vi "Reports.Find Image File Objs Based on Data File Path.vi"(10 "Pattern":string="png", 11 "Data File":path) -> (3 "FIle Objs":T1[](array[typedef]))   [LabVIEW 2018]
uses:
  Report.Result FileDataObject.ctl
  <vilib>/KATE/Files/File Utils.lvlib
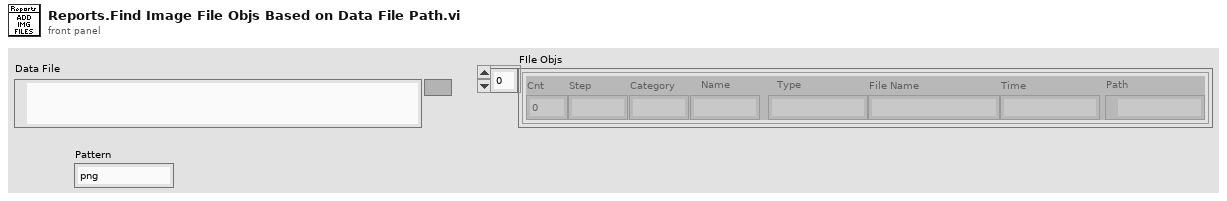
[diagram p1: front panel]
types:
  T1 = typedef "Report.Result FileDataObject.ctl" = cluster{"Cnt":i32, "Step":string, "Category":string, "Name":string, "Type":string, "File Name":string, "Time":string, "Path":path}
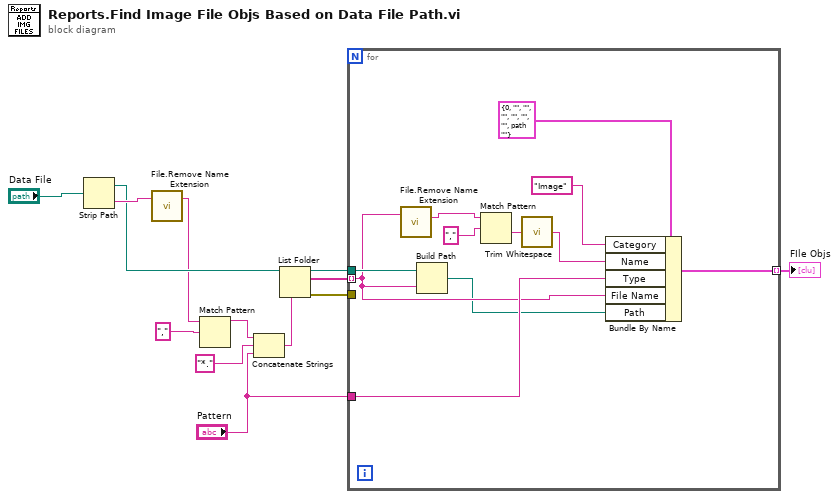
[diagram p0: block diagram]
diagram:
  n1 = Strip Path(path="Data File") -> (stripped path=w12:path, name=w13:string)
  n2 = call <vilib>:"File.Remove Name Extension.vi"("File Name"=w13) -> ("Name Less Ext"=w11:string)  [unwired: 1 in, 1 out]
  n3 = Match Pattern(string=w11, regular expression=",") -> (before substring=w9:string)  [unwired: 1 in, 3 out]
  n4 = Concatenate Strings(w9, "*.", "Pattern") -> (w7:string)
  n5 = List Folder(path=w12, pattern=w7) -> (path out=w5:path, filenames=w4:string[], error out=w1:errorcluster)  [unwired: 2 in, 1 out]
  n6 = for {
    tunnel: w5 -> [w23]
    tunnel: w4 -> [w20] mode=indexing
    tunnel: "Pattern" -> [w21]
    tunnel: [w15] -> w2 mode=indexing
    tunnel: w1 -> [_]
    n7 = call <vilib>:"File.Remove Name Extension.vi"("File Name"=w20) -> ("Name Less Ext"=w18:string)  [unwired: 1 in, 1 out]
    n8 = Build Path(base path=w23, name or relative path=w20) -> (appended path=w14:path)
    n9 = Match Pattern(string=w18, regular expression=",") -> (after substring=w17:string)  [unwired: 1 in, 3 out]
    n10 = call <vilib>:"Trim Whitespace.vi"("string"=w17) -> ("trimmed string"=w16:string)  [unwired: 1 in]
    n11 = Bundle By Name(cluster=T1 {"Cnt"=0, "Step"="", "Category"="", "Name"="", "Type"="", "File Name"="", "Time"="", "Path"=path ""} ("FileData Object"), "Category"="Image", "Name"=w16, "Type"=w21, "File Name"=w20, "Path"=w14) -> (w15:T1)
  }
  "FIle Objs" <- w2
